vi "globals.vi"() -> ()   [LabVIEW 2014]
uses:
  screen-state-machine.ctl
panel:
  out "queue out":refnum<queue>
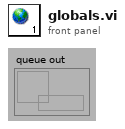
[diagram p1: front panel]
diagram:
